vi "dfd_NStage MRate Get Factors.vi"(6 "filtering mode":T1=2 items=["No Rate Change", "Interpolation", "Decimation"], 8 "error in":errorcluster, 10 "manual factorization":i32[](array[numeric]), 11 "factor":i32=4) -> (0 "error out":errorcluster, 3 "factors":i32[](array[numeric]))   [LabVIEW 2017, in "NI_DigFilterLicensed.lvlib"]
uses:
  <vilib>/addons/Digital Filter Design/NI_DigFilterLicensed.lvlib
  <vilib>/addons/Digital Filter Design/_Objects.llb/DFD Multirate Filtering Mode.ctl
  <vilib>/addons/Digital Filter Design/_Misc.llb/dfd_Error Handlers (Multiple).vi
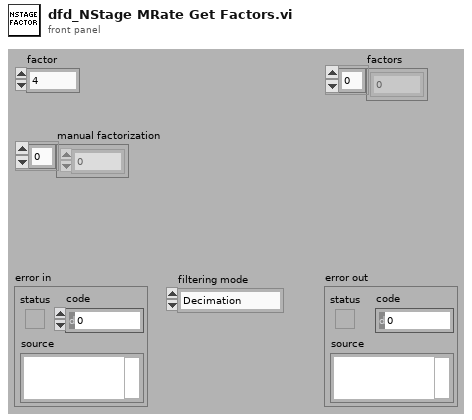
[diagram p1: front panel]
types:
  T1 = typedef "NI_DigFilterLicensed.lvlib/DFD Multirate Filtering Mode.ctl" = u16
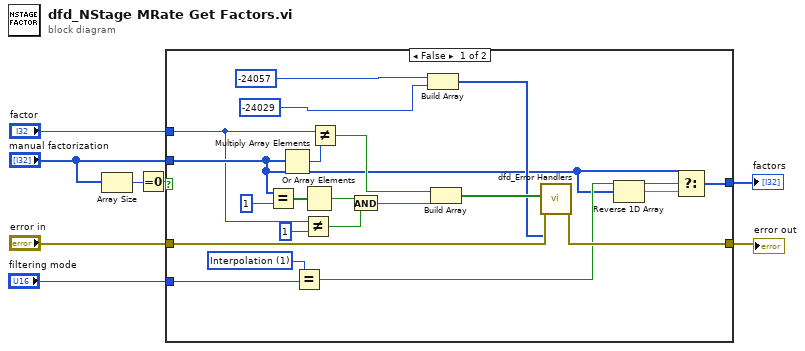
[diagram p0: block diagram]
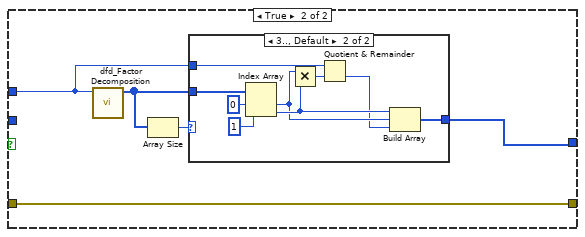
[diagram p2: hidden frame]
diagram:
  n1 = Array Size(array="manual factorization") -> (size(s)=w7:i32)
  n2 = Equal To 0?(x=w7) -> (x = 0?=w8:bool)
  n3 = case shown="False" w8 {
    tunnel: "factor" -> [w13 w33]
    tunnel: "error in" -> [w26 w34]
    tunnel: "manual factorization" -> [w17 _]
    tunnel: [w19 w30] -> w3
    tunnel: [w25 w34] -> w2
    tunnel: "filtering mode" -> [w20 _]
    frame False {
      w15 = T1 1 items=["No Rate Change", "Interpolation", "Decimation"] ("filtering mode")
      n4 = Equal?(x=w17, y=1) -> (x = y?=w24:bool[])
      n5 = Multiply Array Elements(1:w17) -> (0:w29:i32)
      n6 = Equal?(x=w15, y=w20) -> (x = y?=w18:bool)
      n7 = Not Equal?(x=w13, y=1) -> (x != y?=w9:bool)
      n8 = Or Array Elements(Boolean array=w24) -> (logical OR=w10:bool)
      n9 = Not Equal?(x=w13, y=w29) -> (x != y?=w28:bool)
      n10 = And(x=w10, y=w9) -> (x .and. y?=w11:bool)
      n11 = Build Array(-24057 ("ERR_FACOTR_NOT_MATCH"), -24029 ("ERR_#BAND_LE_ONE")) -> (w22:i32[])
      n12 = Build Array(w28, w11) -> (w23:bool[])
      n13 = call-poly <vilib>:"dfd_Error Handlers.vi"("error in (no error)"=w26, "error sources"=w22, "condition failed?"=w23) -> ("error out"=w25:errorcluster)  [unwired: 8 out]
      n14 = Reverse 1D Array(array=w17) -> (reversed array=w16:i32[])
      n15 = Select(t=w17, s=w18, f=w16) -> (s? t:f=w19:i32[])
    }
    frame True {
      n16 = call <vilib>:"dfd_Factor Decomposition.vi"("number"=w33) -> ("factors"=w32:i32[])  [unwired: 10 out]
      n17 = Array Size(array=w32) -> (size(s)=w31:i32)
      n18 = case shown="3.., Default" w31 {
        tunnel: w33 -> [_ w39]
        tunnel: w32 -> [w35 w38]
        tunnel: [w35 w37] -> w30
        frame 1, 2 {
        }
        frame 3.., Default {
          n19 = Index Array(array=w38, index #1=0 ("index"), index #2=1 ("index")) -> (element #1=w40:i32, element #2=w41:i32)
          n20 = Multiply(x=w40, y=w41) -> (x*y=w44:i32)
          n21 = Quotient & Remainder(x=w39, y=w44) -> (floor(x/y)=w36:i32)  [unwired: 1 out]
          n22 = Build Array(w41, w40, w36) -> (w37:i32[])
        }
      }
    }
  }
  "factors" <- w3
  "error out" <- w2
